vi "LDA1_Safety.vi"(1 "Adam Loop Count":i32, 2 "Ch Names":string[](array[string]), 3 "Values":dbl[](array[numeric]) format="%.2f") -> (0 "Scan comment":string)   [LabVIEW 2010]
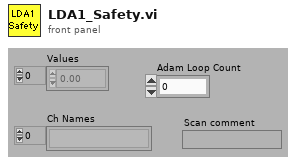
[diagram p1: front panel]
types:
  T1 = typedef "LVDateTimeRec.ctl" = cluster{"fractional second":dbl, "second":i32, "minute":i32, "hour":i32, "day of month":i32, "month":i32, "year":i32, "day of week":i32, "day of year":i32, "DST":i32}
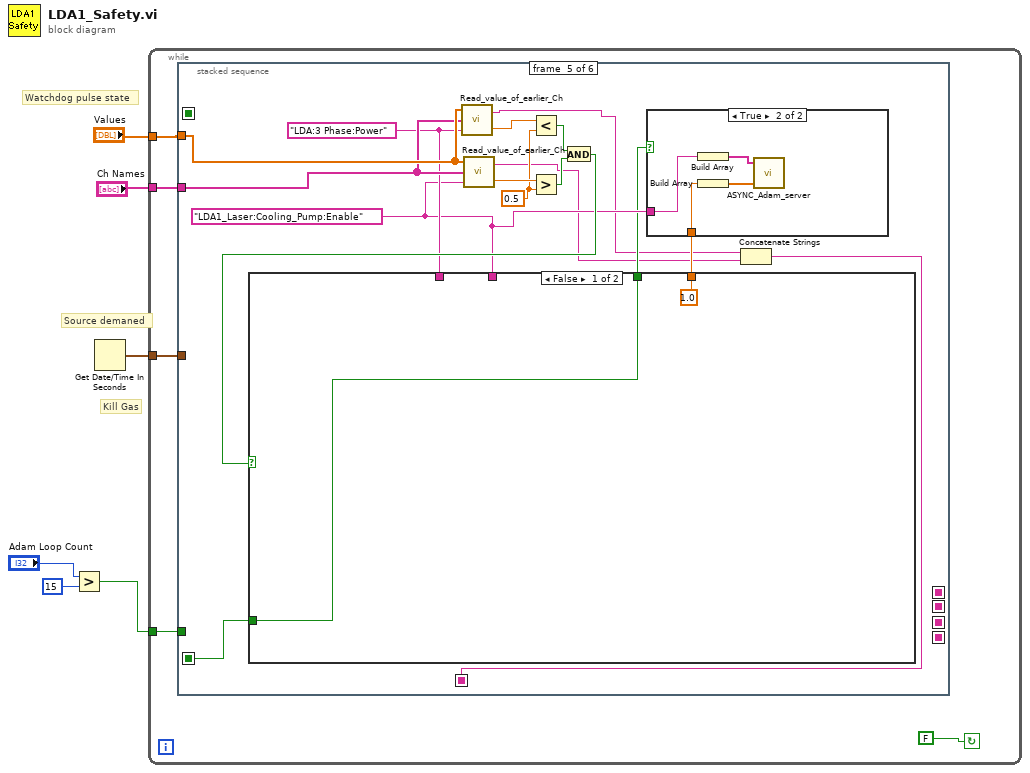
[diagram p0: block diagram]
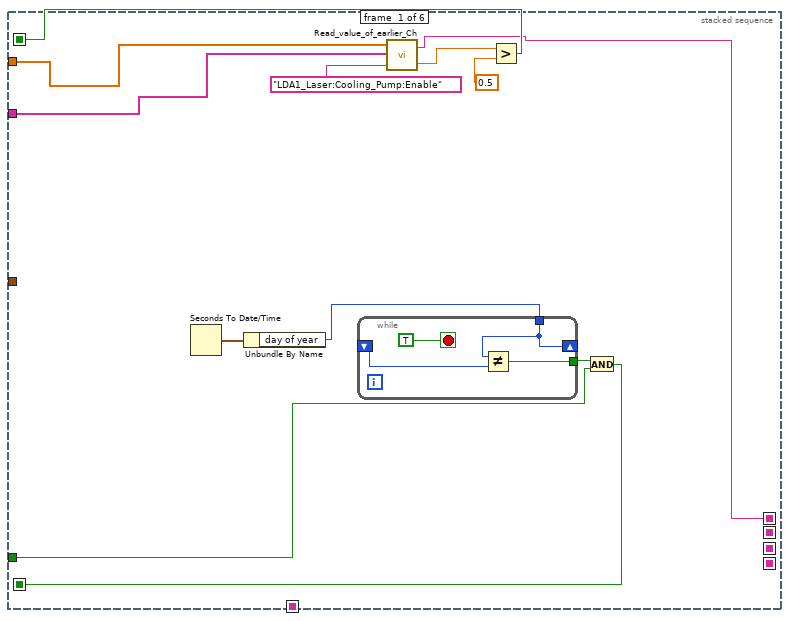
[diagram p2: hidden frame]
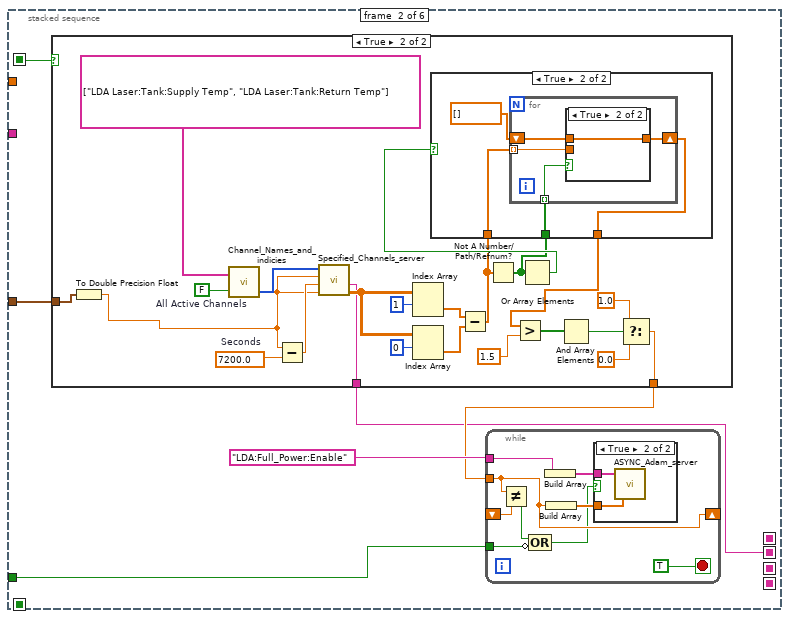
[diagram p3: hidden frame]
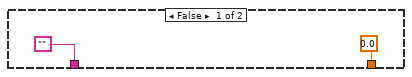
[diagram p5: hidden frame]
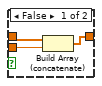
[diagram p7: hidden frame]
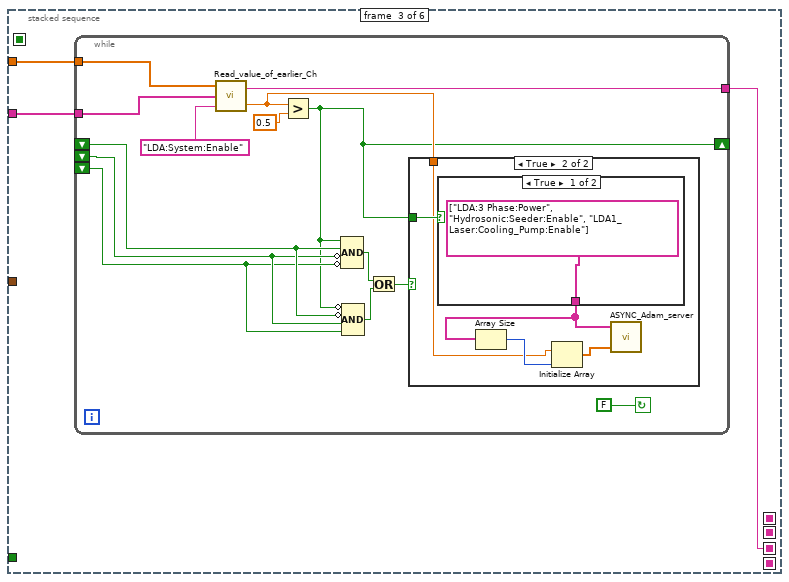
[diagram p8: hidden frame]
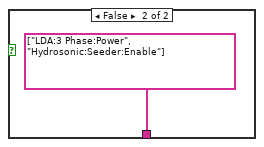
[diagram p10: hidden frame]
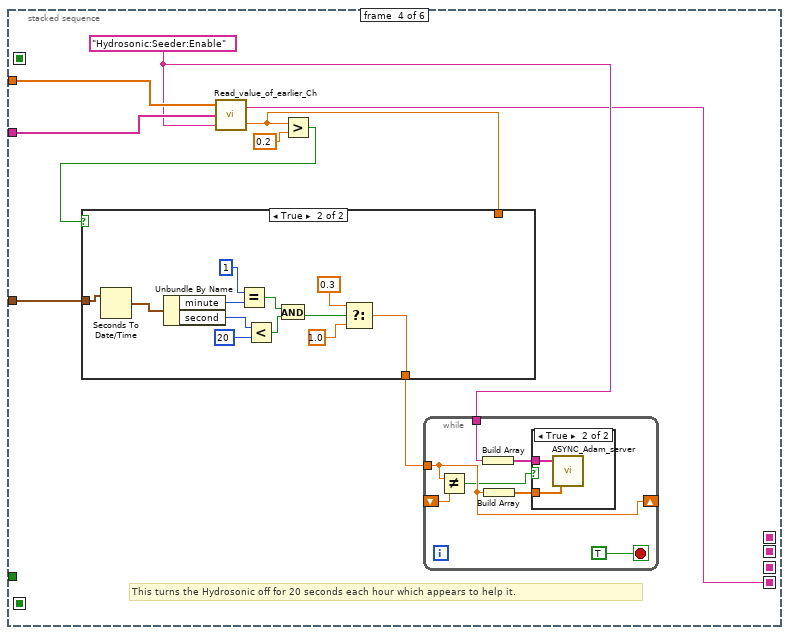
[diagram p11: hidden frame]
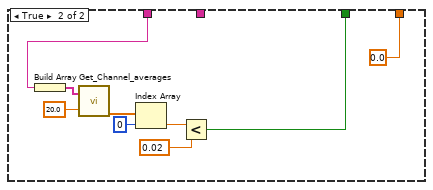
[diagram p15: hidden frame]
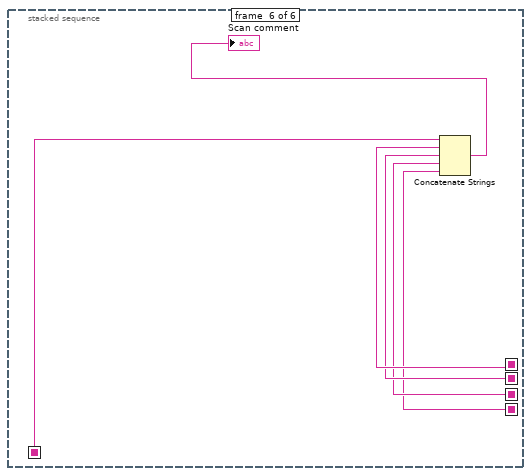
[diagram p16: hidden frame]
diagram:
  # "Source demaned"
  # "Watchdog pulse state"
  # "Kill Gas"
  n1 = Greater?(x="Adam Loop Count", y=15) -> (0:w2:bool)
  n2 = Get Date/Time In Seconds() -> (seconds since 1Jan1904=w1:timestamp)
  n3 = while {
    tunnel: "Ch Names" -> [w11]
    tunnel: "Values" -> [w10]
    tunnel: w2 -> [w8]
    tunnel: w1 -> [w7]
    stop <- FALSE continue-if-true
    n4 = stacked-sequence {
      seq-local: [w13 _ _ _ _ _] -> [_ _ _ _ w141 _]
      seq-local: [w21 _ _ _ _ _] -> [_ w32 _ _ _ _]
      seq-local: [w17 _ _ _ _ _] -> [_ _ _ _ _ w174]
      seq-local: [_ w28 _ _ _ _] -> [_ _ _ _ _ w173]
      seq-local: [_ _ w83 _ _ _] -> [_ _ _ _ _ w172]
      seq-local: [_ _ _ w107 _ _] -> [_ _ _ _ _ w171]
      seq-local: [_ _ _ _ w138 _] -> [_ _ _ _ _ w169]
      tunnel: w11 -> [w22 _ w84 w114 w151 _]
      tunnel: w10 -> [w23 _ w85 w115 w152 _]
      tunnel: w8 -> [w12 w30 _ _ _ _]
      tunnel: w7 -> [_ w33 _ w110 _ _]
      frame #0 {
        n5 = Seconds To Date/Time() -> (date time rec=w16:T1)  [unwired: 2 in]
        n6 = Unbundle By Name(w16) -> ("day of year"=w15:i32)
        n7 = while {
          shift-right: [w27] -> _
          shift-left: _ -> [w26]
          tunnel: w15 -> [w27]
          tunnel: [w25] -> w14
          stop <- TRUE stop-if-true
          n8 = Not Equal?(x=w27, y=w26) -> (x != y?=w25:bool)
        }
        n9 = call "Read_value_of_earlier_Ch.vi"("Desired Ch to Read"="LDA1_Laser:Cooling_Pump:Enable", "Ch names"=w22, "Present scan array"=w23) -> ("Value"=w19:dbl, "Scan comment"=w17:string)  [unwired: 1 in]
        n10 = Greater?(x=w19, y=0.5) -> (0:w21:bool)
        n11 = And(x=w14, y=w12) -> (x .and. y?=w13:bool)
      }
      frame #1 {
        n12 = case shown="True" w32 {
          tunnel: w33 -> [_ w69]
          tunnel: [0.0 ("y") w54] -> w29
          tunnel: ["" w47] -> w28
          frame False {
          }
          frame True {
            w67 = 7200.0  # Seconds
            w65 = FALSE  # All Active Channels
            n13 = To Double Precision Float(number=w69) -> (double precision float=w63:dbl)
            n14 = call "Channel_Names_and_indicies.vi"("All Active Channels"=w65, "Desired Ch Names"=string[] ["LDA Laser:Tank:Supply Temp", "LDA Laser:Tank:Return Temp"]) -> ("Indicies"=w66:i32[])  [unwired: 1 out]
            n15 = Subtract(x=w63, y=w67) -> (x-y=w68:dbl)
            n16 = call "Specified_Channels_server.vi"("End time"=w63, "Start time"=w68, "Clients time"=w63, "Requested channels"=w66) -> ("Output array"=w60:dbl[][], "Messages"=w47:string)  [unwired: 1 in, 3 out]
            n17 = Index Array(array=w60, index (row)=1) -> (element=w59:dbl[])  [unwired: 1 in]
            n18 = Index Array(array=w60, index (row)=0) -> (element=w58:dbl[])  [unwired: 1 in]
            n19 = Subtract(x=w59, y=w58) -> (x-y=w49:dbl[])
            n20 = Not A Number/Path/Refnum?(number/path/refnum=w49) -> (NaN/Path/Refnum?=w50:bool[])
            n21 = Or Array Elements(Boolean array=w50) -> (logical OR=w51:bool)
            n22 = case shown="True" w51 {
              tunnel: w50 -> [_ w74]
              tunnel: w49 -> [w70 w73]
              tunnel: [w70 w71] -> w48
              frame False {
              }
              frame True {
                n23 = for {
                  shift-right: [w77] -> w71
                  shift-left: dbl[] [] -> [w76]
                  tunnel: w74 -> [w78] mode=indexing
                  tunnel: w73 -> [w75] mode=indexing
                  n24 = case shown="True" w78 {
                    tunnel: [w80 w82] -> w77
                    tunnel: w76 -> [w81 w82]
                    tunnel: w75 -> [w79 _]
                    frame False {
                      n25 = Build Array (concatenate)(w81, w79) -> (w80:dbl[])
                    }
                    frame True {
                    }
                  }
                }
              }
            }
            n26 = Greater?(x=w48, y=1.5) -> (0:w53:bool[])
            n27 = And Array Elements(Boolean array=w53) -> (logical AND=w52:bool)
            n28 = Select(t=1.0 ("y"), s=w52, f=0.0 ("y")) -> (s? t:f=w54:dbl)
          }
        }
        n29 = while {
          shift-right: [w38] -> _
          shift-left: _ -> [w39]
          tunnel: w29 -> [w38]
          tunnel: "LDA:Full_Power:Enable" -> [w40]
          tunnel: w30 -> [w35]
          stop <- TRUE stop-if-true
          n30 = Not Equal?(x=w38, y=w39) -> (x != y?=w36:bool)
          n31 = Compound Arithmetic op=OR(w36, invert w35) -> (w34:bool)
          n32 = Build Array(w40) -> (w41:string[])
          n33 = Build Array(w38) -> (w42:dbl[])
          n34 = case shown="True" w34 {
            tunnel: w42 -> [_ w44]
            tunnel: w41 -> [_ w43]
            frame False {
            }
            frame True {
              n35 = call "ASYNC_Adam_server.vi"("Values"=w44, "Channel Names"=w43) -> ()  [unwired: 1 in, 3 out]
            }
          }
        }
      }
      frame #2 {
        n36 = while {
          tunnel: w85 -> [w99]
          tunnel: w84 -> [w98]
          shift-right: [w87] -> _
          shift-left: _ -> [w93]
          shift-left: _ -> [w92]
          shift-left: _ -> [w91]
          tunnel: [w86] -> w83
          stop <- FALSE continue-if-true
          n37 = call "Read_value_of_earlier_Ch.vi"("Desired Ch to Read"="LDA:System:Enable", "Ch names"=w98, "Present scan array"=w99) -> ("Value"=w94:dbl, "Scan comment"=w86:string)  [unwired: 1 in]
          n38 = Greater?(x=w94, y=0.5) -> (0:w87:bool)
          n39 = Compound Arithmetic op=AND(w87, w93, invert w92, invert w91) -> (w89:bool)
          n40 = Compound Arithmetic op=AND(invert w87, invert w93, w92, w91) -> (w90:bool)
          n41 = Or(x=w89, y=w90) -> (x .or. y?=w88:bool)
          n42 = case shown="True" w88 {
            tunnel: w94 -> [_ w100]
            tunnel: w87 -> [_ w104]
            frame False {
            }
            frame True {
              n43 = case shown="True" w104 {
                tunnel: [string[] ["LDA:3 Phase:Power", "Hydrosonic:Seeder:Enable", "LDA1_Laser:Cooling_Pump:Enable"] ("Channel Names") string[] ["LDA:3 Phase:Power", "Hydrosonic:Seeder:Enable"] ("Channel Names")] -> w103
                frame True {
                }
                frame False {
                }
              }
              n44 = Array Size(array=w103) -> (size(s)=w101:i32)
              n45 = Initialize Array(w100, w101) -> (w102:dbl[])
              n46 = call "ASYNC_Adam_server.vi"("Values"=w102, "Channel Names"=w103) -> ()  [unwired: 1 in, 3 out]
            }
          }
        }
      }
      frame #3 {
        w109 = "Hydrosonic:Seeder:Enable" ("Desired Ch to Read")
        # "This turns the Hydrosonic off for 20 seconds each hour which appears to help it."
        n47 = call "Read_value_of_earlier_Ch.vi"("Desired Ch to Read"=w109, "Ch names"=w114, "Present scan array"=w115) -> ("Value"=w112:dbl, "Scan comment"=w107:string)  [unwired: 1 in]
        n48 = Greater?(x=w112, y=0.2) -> (0:w111:bool)
        n49 = case shown="True" w111 {
          tunnel: w112 -> [w125 _]
          tunnel: w110 -> [_ w136]
          tunnel: [w125 w126] -> w108
          frame False {
          }
          frame True {
            n50 = Seconds To Date/Time(time stamp (now)=w136) -> (date time rec=w137:T1)  [unwired: 1 in]
            n51 = Unbundle By Name(w137) -> ("minute"=w135:i32, "second"=w133:i32)
            n52 = Equal?(x=1, y=w135) -> (x = y?=w130:bool)
            n53 = Less?(x=w133, y=20) -> (x < y?=w131:bool)
            n54 = And(x=w130, y=w131) -> (x .and. y?=w129:bool)
            n55 = Select(t=0.3 ("y"), s=w129, f=1.0) -> (s? t:f=w126:dbl)
          }
        }
        n56 = while {
          shift-right: [w118] -> _
          shift-left: _ -> [w119]
          tunnel: w108 -> [w118]
          tunnel: w109 -> [w120]
          stop <- TRUE stop-if-true
          n57 = Not Equal?(x=w118, y=w119) -> (x != y?=w116:bool)
          n58 = Build Array(w120) -> (w121:string[])
          n59 = Build Array(w118) -> (w122:dbl[])
          n60 = case shown="True" w116 {
            tunnel: w122 -> [_ w124]
            tunnel: w121 -> [_ w123]
            frame False {
            }
            frame True {
              n61 = call "ASYNC_Adam_server.vi"("Values"=w124, "Channel Names"=w123) -> ()  [unwired: 1 in, 3 out]
            }
          }
        }
      }
      frame #4 {
        w145 = "LDA:3 Phase:Power" ("Desired Ch to Read")
        w150 = 0.5 ("y")
        w144 = "LDA1_Laser:Cooling_Pump:Enable" ("Desired Ch to Read")
        n62 = call "Read_value_of_earlier_Ch.vi"("Desired Ch to Read"=w145, "Ch names"=w151, "Present scan array"=w152) -> ("Value"=w149:dbl, "Scan comment"=w140:string)  [unwired: 1 in]
        n63 = call "Read_value_of_earlier_Ch.vi"("Desired Ch to Read"=w144, "Ch names"=w151, "Present scan array"=w152) -> ("Value"=w153:dbl, "Scan comment"=w139:string)  [unwired: 1 in]
        n64 = Less?(x=w149, y=w150) -> (x < y?=w148:bool)
        n65 = Greater?(x=w153, y=w150) -> (0:w147:bool)
        n66 = And(x=w148, y=w147) -> (x .and. y?=w146:bool)
        n67 = case shown="False" w146 {
          tunnel: w145 -> [_ w162]
          tunnel: w144 -> [_ _]
          tunnel: [w158 w161] -> w143
          tunnel: [1.0 ("element") 0.0 ("element")] -> w142
          tunnel: w141 -> [w158 _]
          frame False {
          }
          frame True {
            n68 = Build Array(w162) -> (w167:string[])
            n69 = call "Get_Channel_averages.vi"("Desired Ch Names"=w167, "Averaging time (mins)"=20.0) -> ("number"=w166:dbl[])  [unwired: 1 in, 2 out]
            n70 = Index Array(array=w166, index=0) -> (element=w164:dbl)
            n71 = Less?(x=w164, y=0.02) -> (x < y?=w161:bool)
          }
        }
        n72 = case shown="True" w143 {
          tunnel: w144 -> [_ w155]
          tunnel: w142 -> [_ w154]
          frame False {
          }
          frame True {
            n73 = Build Array(w155) -> (w156:string[])
            n74 = Build Array(w154) -> (w157:dbl[])
            n75 = call "ASYNC_Adam_server.vi"("Values"=w157, "Channel Names"=w156) -> ()  [unwired: 1 in, 3 out]
          }
        }
        n76 = Concatenate Strings(w140, w139) -> (w138:string)
      }
      frame #5 {
        n77 = Concatenate Strings(w169, w174, w173, w172, w171) -> (→"Scan comment":string)
      }
    }
  }
